vi "Create Framework Configuration.vi"(11 "Plugins":T4(array[cluster])=[{"plugin class"="udp", "channel count per transfer"=100, "transfer configs per group"=[], "group configs"=[], "plugin timing"={"Decimation"=1, "Offset"=0}}]) -> (3 "Framework Configuration":T5)   [LabVIEW 2017]
uses:
  Source/Shared/Typedefs/DSF.Shared.Refactor.Typedefs.Framework Configuration.Aggregate.ctl
  Source/Shared/Typedefs/DSF.Shared.Refactor.Typedefs.Plugin Configuration.Aggregate.ctl
  Source/Shared/Typedefs/DSF.Shared.Typedefs.Cycle Timing Factors.ctl
  Source/Shared/Typedefs/DSF.Shared.Refactor.Typedefs.Transfer Group Configuration.Aggregate.ctl
  Source/Shared/Typedefs/DSF.Shared.Typedefs.Direction.ctl
  Source/Shared/Typedefs/DSF.Shared.Refactor.Typedefs.Transfer Configuration.ctl
  Source/Shared/Typedefs/DSF.Shared.Typedefs.Byte Order.ctl
  Source/Shared/Typedefs/DSF.Shared.Refactor.Typedefs.Channel Array Configuration.ctl
  Source/Shared/Typedefs/DSF.Shared.Typedefs.Data Type.ctl
  Source/DSF.Shared.lvlib
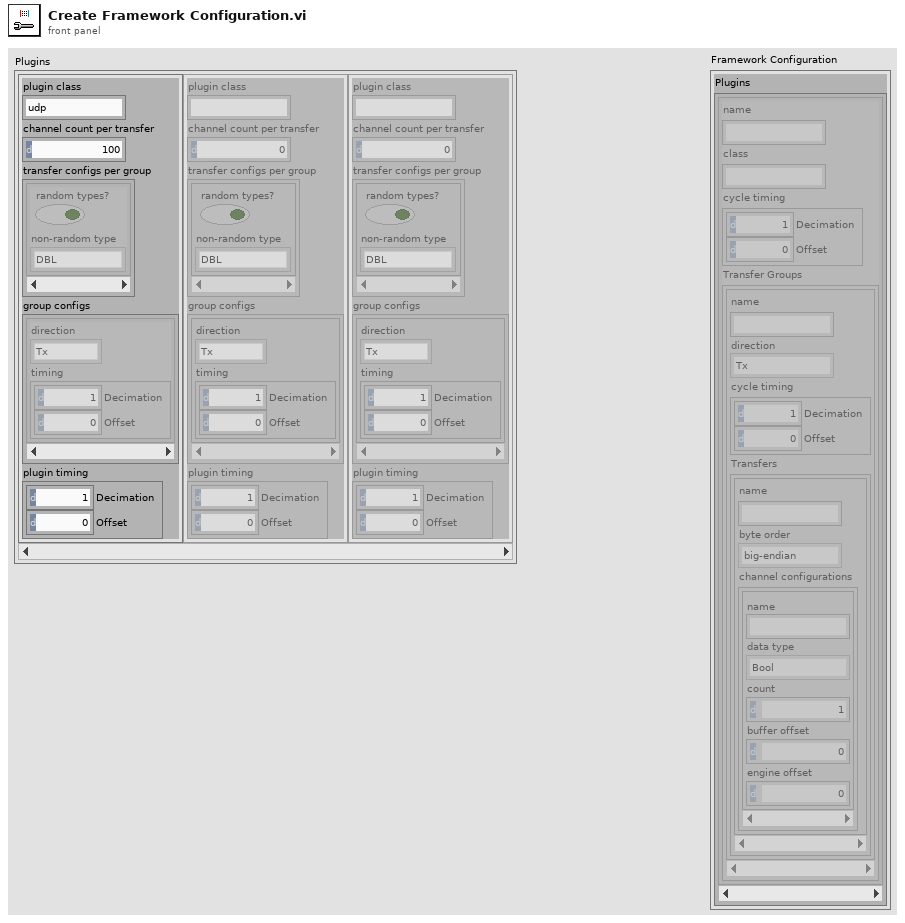
[diagram p1: front panel]
types:
  T1 = typedef "DSF.Shared.lvlib/DSF.Shared.Typedefs.Data Type.ctl" = enum8{"Bool", "SGL", "DBL", "I8", "I16", "I32", "I64", "U8", "U16", "U32", "U64"}
  T2 = typedef "DSF.Shared.lvlib/DSF.Shared.Typedefs.Direction.ctl" = enum8{"Tx", "Rx"}
  T3 = typedef "DSF.Shared.lvlib/DSF.Shared.Typedefs.Cycle Timing Factors.ctl" = cluster{"Decimation":u64, "Offset":u64}
  T4 = cluster{"plugin class":string, "channel count per transfer":i32, "transfer configs per group":cluster{"random types?":bool, "non-random type":T1}[], "group configs":cluster{"direction":T2, "timing":T3}[], "plugin timing":T3}[]
  T5 = typedef "DSF.Shared.lvlib/DSF.Shared.Refactor.Typedefs.Framework Configuration.Aggregate.ctl" = cluster{"Plugins":T6[]}
  T6 = typedef "DSF.Shared.lvlib/DSF.Shared.Refactor.Typedefs.Plugin Configuration.Aggregate.ctl" = cluster{"name":string, "class":string, "cycle timing":T3, "Transfer Groups":T7[]}
  T7 = typedef "DSF.Shared.lvlib/DSF.Shared.Refactor.Typedefs.Transfer Group Configuration.Aggregate.ctl" = cluster{"name":string, "direction":T2, "cycle timing":T3, "Transfers":T8[]}
  T8 = typedef "DSF.Shared.lvlib/DSF.Shared.Refactor.Typedefs.Transfer Configuration.ctl" = cluster{"name":string, "byte order":T9, "channel configurations":T10[]}
  T9 = typedef "DSF.Shared.lvlib/DSF.Shared.Typedefs.Byte Order.ctl" = enum8{"big-endian", "little-endian"}
  T10 = typedef "DSF.Shared.lvlib/DSF.Shared.Refactor.Typedefs.Channel Array Configuration.ctl" = cluster{"name":string, "data type":T1, "count":u64, "buffer offset":u64, "engine offset":u64}
  T11 = cluster{"random types?":bool, "non-random type":T1}[]
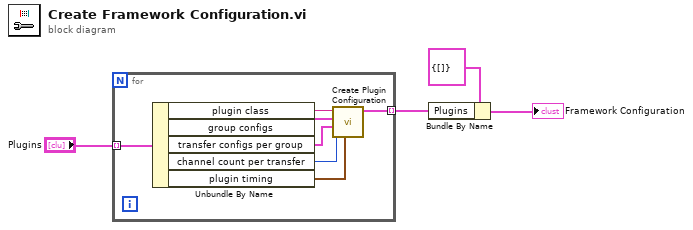
[diagram p0: block diagram]
diagram:
  n1 = for {
    tunnel: [w11] -> w3 mode=indexing
    tunnel: "Plugins" -> [w10] mode=indexing
    n2 = Unbundle By Name(w10) -> ("plugin class"=w9:string, "group configs"=w7:cluster{"direction":T2, "timing":T3}[], "transfer configs per group"=w5:T11, "channel count per transfer"=w6:i32, "plugin timing"=w8:T3)
    n3 = call "Create Plugin Configuration.vi"("plugin timing"=w8, "channel count per transfer"=w6, "transfer configs"=w5, "group configs"=w7, "plugin class"=w9) -> ("plugin configuration"=w11:T6)  [unwired: 6 in]
  }
  n4 = Bundle By Name(cluster=T5 {"Plugins"=[]} ("Framework Configuration"), "Plugins"=w3) -> (→"Framework Configuration":T5)
